vi "Preview LastElement.vi"(8 "error in":errorcluster, 11 "Buffer in":refnum<data-value>) -> (0 "error out":errorcluster, 1 "found":bool, 2 "element":variant, 3 "Buffer":refnum<data-value>)   [LabVIEW 2013, in "VariantBuffer.lvclass"]
doc: "This VI returns data from the ring buffer starting from the oldest data and ending with the newest.\n\nThe data is duplicated at the output so this VI allocates new place in the memory for the output."
uses:
  VariantBuffer.lvclass
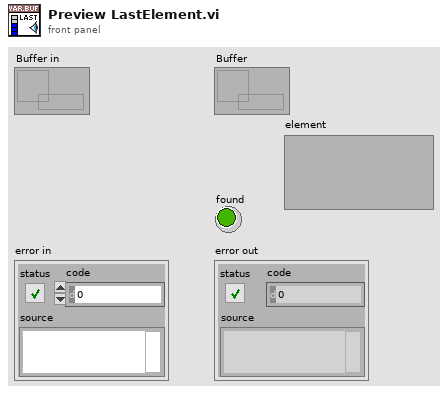
[diagram p1: front panel]
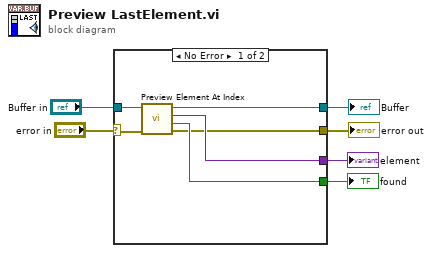
[diagram p0: block diagram]
diagram:
  n1 = case shown="No Error" "error in" {
    selector: "error in" -> [w8 w13]
    tunnel: "Buffer in" -> [w12 w14]
    tunnel: [w11 w14] -> w6
    tunnel: [w7 w13] -> w3
    tunnel: [w10 _] -> w5
    tunnel: [w9 _] -> w2
    frame No Error {
      n2 = call "Preview Element At Index.vi"("error in"=w8, "Buffer in"=w12) -> ("error out"=w7:errorcluster, "found"=w9:bool, "element"=w10:variant, "Buffer"=w11:refnum<data-value>)  [unwired: 6 in]
    }
    frame Error {
    }
  }
  "error out" <- w3
  "Buffer" <- w6
  "element" <- w5
  "found" <- w2
